vi "Set TimerState.vi"(6 "State (On/Off)":bool, 7 "Timer Number":T1, 8 "error in (no error)":errorcluster, 10 "Address (0)":i32, 11 "VISA resource name":refnum<visa-resource-name>) -> (0 "error out":errorcluster, 3 "VISA resource name out":refnum<visa-resource-name>)   [LabVIEW 2016, in "Environment Chamber.lvlib" / "Climatic Chamber.lvlib"]
doc: "<b>Valid timer setting</b>\n\nStarts or stops the specified timer."
uses:
  Climatic Chamber.lvlib
  Private/Type Defs/TimerNumber Enum.ctl
panel:
  out "NACK":bool
  out "Error":bool
  out "ACK":bool
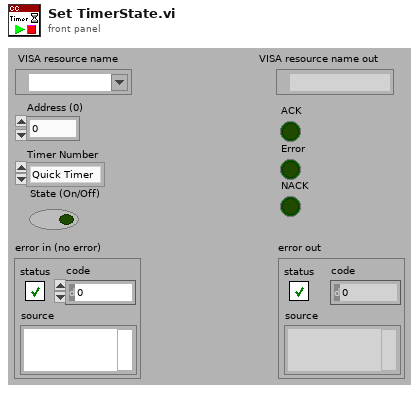
[diagram p1: front panel]
types:
  T1 = typedef "Environment Chamber.lvlib/Climatic Chamber.lvlib/TimerNumber Enum.ctl" = enum16{"Quick Timer", "Start Timer", "End Timer"}
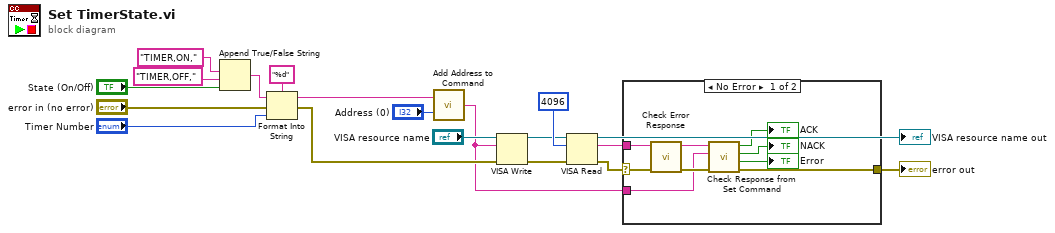
[diagram p0: block diagram]
diagram:
  n1 = Append True/False String(1:"State (On/Off)", 2:"TIMER,OFF,", 3:"TIMER,ON,") -> (0:w1:string)  [unwired: 1 in]
  n2 = Format Into String(format string="%d", initial string=w1, error in="error in (no error)", "Timer Number") -> (resulting string=w8:string, error out=w19:errorcluster)
  n3 = call "Add Address to Command.vi"("Address (0)"="Address (0)", "Command"=w8) -> ("Command OUT"=w9:string)
  n4 = VISA Write(VISA resource name="VISA resource name", write buffer=w9, error in (no error)=w19) -> (VISA resource name out=w16:refnum<visa-resource-name>, error out=w15:errorcluster)  [unwired: 1 out]
  n5 = VISA Read(VISA resource name=w16, byte count=u32 4096, error in (no error)=w15) -> (VISA resource name out=→"VISA resource name out":refnum<visa-resource-name>, read buffer=w11:string, error out=w12:errorcluster)  [unwired: 1 out]
  n6 = case shown="No Error" w12 {
    selector: w12 -> [w27 w29]
    tunnel: w11 -> [w28 _]
    tunnel: [w23 w29] -> w10
    tunnel: w9 -> [w24 _]
    frame No Error {
      n7 = call "Check Error Response.vi"("error in (no error)"=w27, "read String"=w28) -> ("error out"=w26:errorcluster, "String out"=w25:string)  [unwired: 7 in, 1 out]
      n8 = call "Check Response from Set Command.vi"("error in (no error)"=w26, "Command"=w24, "Response"=w25) -> ("error out"=w23:errorcluster, "Error"=→"Error":bool, "NACK"=→"NACK":bool, "ACK"=→"ACK":bool)  [unwired: 5 in]
    }
    frame Error {
    }
  }
  "error out" <- w10
